vi "Global variable.vi"() -> ()   [LabVIEW 2024]
panel:
  in  "leak data":string
  in  "marking Data":string
  in  "MArking Complete":bool
  in  "Exit":bool
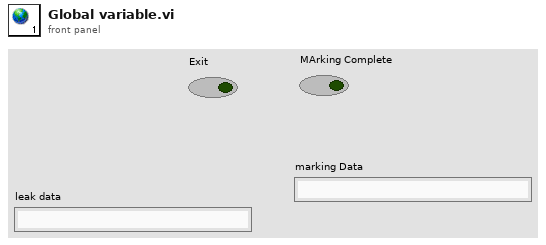
[diagram p1: front panel]
diagram:
